vi "Create PINGREQ Packet.vi"(5 "PINGREQ in":refnum<class "PINGREQ.lvclass">, 8 "error in (no error)":errorcluster) -> (0 "error out":errorcluster, 3 "PINGREQ out":refnum<class "PINGREQ.lvclass">)   [LabVIEW 2013, in "MQTT_Control_Packets.lvlib" / "PINGREQ.lvclass"]
uses:
  PINGREQ.lvclass
  ControlPacket/ControlPacket.lvclass/ControlPacket.ctl
  ControlPacket/ControlPacket.lvclass
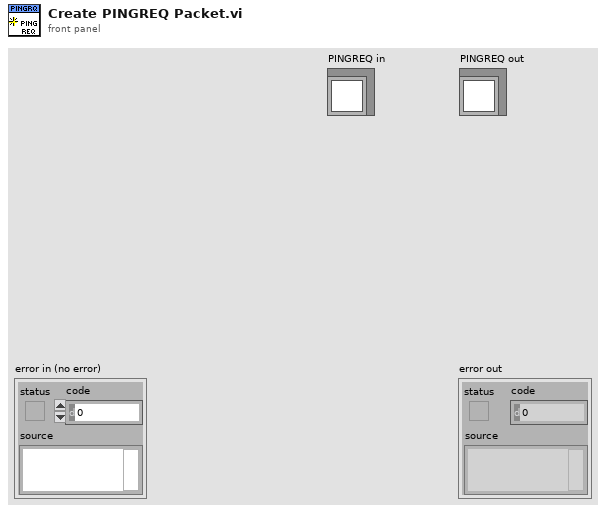
[diagram p1: front panel]
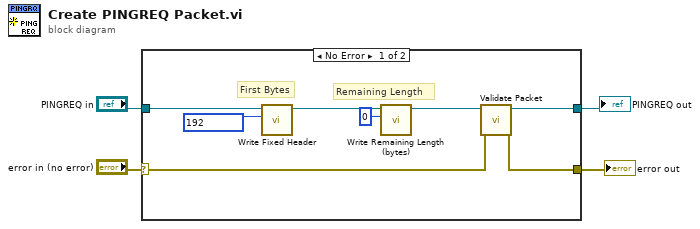
[diagram p0: block diagram]
diagram:
  n1 = case shown="No Error" "error in (no error)" {
    selector: "error in (no error)" -> [w6 w14]
    tunnel: [w5 w14] -> w1
    tunnel: [w7 w13] -> w2
    tunnel: "PINGREQ in" -> [w12 w13]
    frame No Error {
      # "Remaining Length"
      # "First Bytes"
      n2 = call "Write Fixed Header.vi"("Fixed Header"=u8 192, "ControlPacket in"=w12) -> ("ControlPacket out"=w11:refnum<class "PINGREQ.lvclass">)  [unwired: 9 in]
      n3 = call "Write Remaining Length (bytes).vi"("Remaining Length (bytes)"=u32 0, "ControlPacket in"=w11) -> ("ControlPacket out"=w8:refnum<class "PINGREQ.lvclass">)  [unwired: 9 in]
      n4 = call "Validate Packet.vi"("error in (no error)"=w6, "ControlPacket in"=w8) -> ("error out"=w5:errorcluster, "ControlPacket out"=w7:refnum<class "PINGREQ.lvclass">)  [unwired: 8 in]
    }
    frame Error {
    }
  }
  "error out" <- w1
  "PINGREQ out" <- w2
